vi "GetTestVariables.vi"(8 "error in (no error)":errorcluster, 11 "reference in":refnum<class "Driver_Template.lvclass">) -> (0 "error out":errorcluster, 2 "TestVariables":variant[](array[variant]), 3 "reference out":refnum<class "Driver_Template.lvclass">)   [LabVIEW 2014]
uses:
  Driver_Template.lvclass
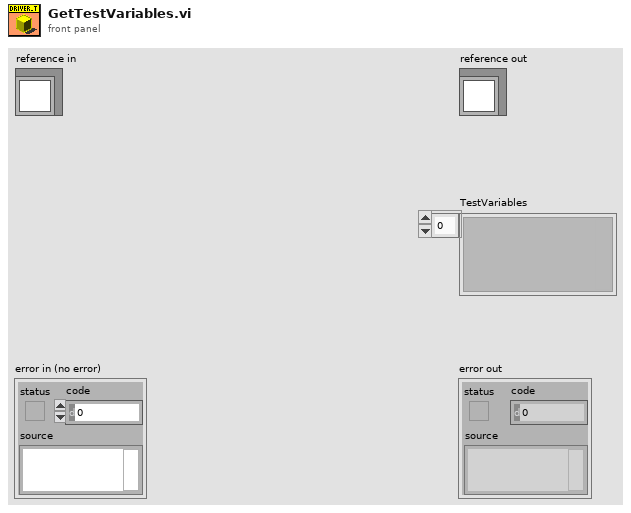
[diagram p1: front panel]
types:
  T1 = typedef "Driver_Template.lvlib/Driver_Template.lvclass/ObjectAttributes.ctl" = cluster{"Config":T2}
  T2 = typedef "Driver_Template.lvlib/Driver_Template.lvclass/Config.ctl" = cluster{"default":string}
  T3 = typedef "Driver_Template.lvlib/Driver_Template.lvclass/TestVariables.ctl" = cluster{"Var1":dbl}
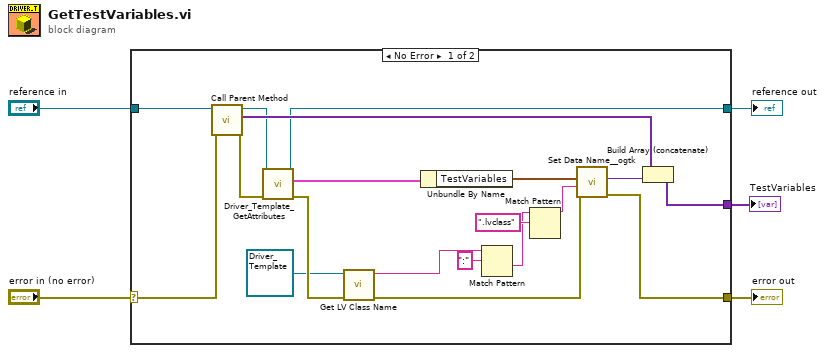
[diagram p0: block diagram]
diagram:
  n1 = case shown="No Error" "error in (no error)" {
    selector: "error in (no error)" -> [w24 w26]
    tunnel: [w13 w26] -> w4
    tunnel: [w6 w25] -> w2
    tunnel: "reference in" -> [w23 w25]
    tunnel: [w17 _] -> w1
    frame No Error {
      n2 = call-parent "Call Parent Method"("error in (no error)"=w24, "ViKing_Base in"=w23) -> ("error out"=w22:errorcluster, "TestVariables"=w18:variant[], "ViKing_Base out"=w7:refnum<class "Driver_Template.lvclass">)  [unwired: 7 in]
      n3 = call "Driver_Template_GetAttributes.vi"("error in (no error)"=w22, "reference in"=w7) -> ("error out"=w16:errorcluster, "Data"=w21:T1, "reference out"=w6:refnum<class "Driver_Template.lvclass">)  [unwired: 6 in, 1 out]
      n4 = call <vilib>:"Get LV Class Name.vi"("error in (no error)"=w16, "object"=refnum<class "Driver_Template.lvclass"> refnum ("ViKing_Base out")) -> ("error out"=w14:errorcluster, "class name"=w12:string)  [unwired: 8 in]
      n5 = Unbundle By Name(w21) -> ("TestVariables"=w20:T3)
      n6 = Match Pattern(string=w12, regular expression=":") -> (after substring=w9:string)  [unwired: 1 in, 3 out]
      n7 = Match Pattern(string=w9, regular expression=".lvclass") -> (before substring=w8:string)  [unwired: 1 in, 3 out]
      n8 = call <userlib>:"Set Data Name__ogtk.vi"("error in (no error)"=w14, "Data Name"=w8, "Data"=w20) -> ("error out"=w13:errorcluster, "Renamed Data"=w19:variant)  [unwired: 7 in]
      n9 = Build Array (concatenate)(w18, w19) -> (w17:variant[])
    }
    frame Error {
    }
  }
  "error out" <- w4
  "reference out" <- w2
  "TestVariables" <- w1
